vi "test Read Message (TCP) Retries Until Success.vi"(8 "error in (no error)":errorcluster, 11 "TestCase in":refnum<class "TCP API Tests.lvclass">) -> (0 "error out":errorcluster, 3 "TestCase out":refnum<class "TCP API Tests.lvclass">)   [LabVIEW 2013, in "TCP API Tests.lvclass"]
uses:
  TCP API Tests.lvclass
  vi.lib/NI/STM/TCP/TCP Data Info.ctl
  vi.lib/NI/STM/TCP/TCP Read Options.ctl
  vi.lib/NI/STM/TCP/TCP Write Options.ctl
  vi.lib/NI/STM/TCP/Write Meta Data (TCP Ref).vi
  vi.lib/NI/STM/TCP/Read Meta Data (TCP Ref).vi
  vi.lib/NI/STM/TCP/Write Message (TCP).vi
  vi.lib/NI/STM/TCP/Write Meta Data (TCP Clst).vi
  vi.lib/NI/STM/TCP/Read Meta Data (TCP Clst).vi
  vi.lib/NI/STM/TCP/Read Message (TCP).vi
  <vilib>/addons/_JKI Toolkits/VI Tester/TestCase.llb/TestCase.lvclass
  vi.lib/NI/STM/NI STM.lvlib
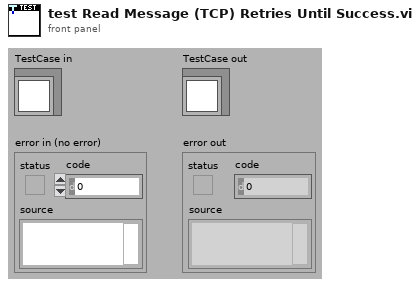
[diagram p1: front panel]
types:
  T1 = typedef "NI STM.lvlib/TCP Data Info.ctl" = cluster{"data size":i32, "retry read":bool}
  T2 = typedef "NI STM.lvlib/TCP Read Options.ctl" = cluster{"ignore timeout error":bool, "timeout ms (1000)":i32}
  T3 = typedef "NI STM.lvlib/TCP Write Options.ctl" = cluster{"ignore timeout error":bool, "timeout ms (1000)":i32}
  T4 = typedef "NI STM.lvlib/TCP Connection Info.ctl" = cluster{"connection ID":refnum<k5>, "meta data":T5[]}
  T5 = typedef "NI STM.lvlib/MetaDataElement.ctl" = string
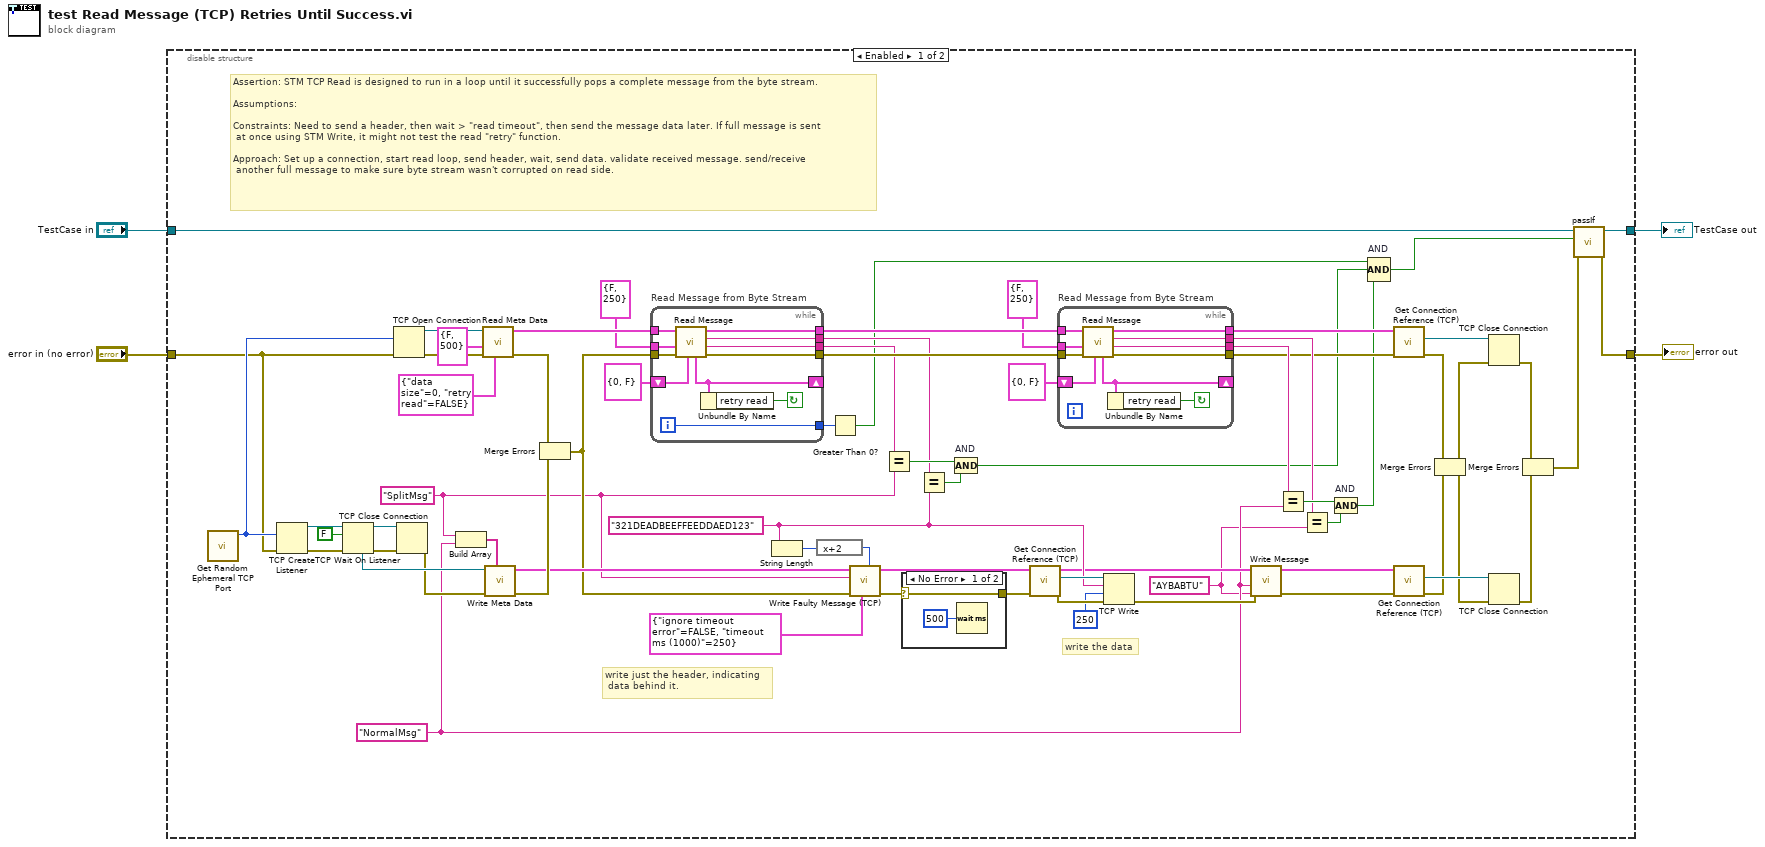
[diagram p0: block diagram]
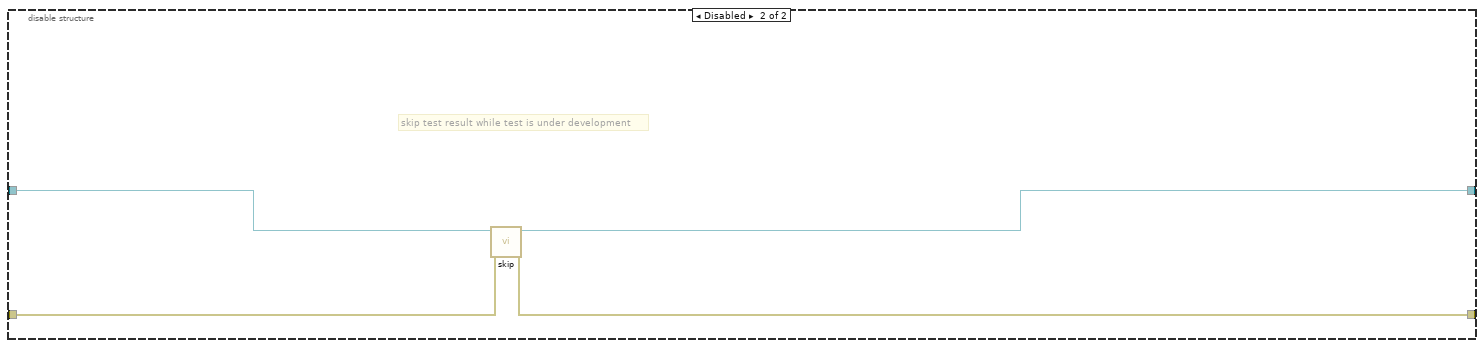
[diagram p3: hidden frame]
diagram:
  n1 = disable-structure shown="Enabled" {
    disable-tunnel: "TestCase in" -> [w72 w100]
    disable-tunnel: [w71 w98] -> w1
    disable-tunnel: [w70 w99] -> w3
    disable-tunnel: "error in (no error)" -> [w56 w97]
    frame Enabled {
      w25 = "AYBABTU" ("data")
      w26 = "NormalMsg" ("Meta Element")
      w39 = "321DEADBEEFFEEDDAED123"
      w40 = "SplitMsg" ("Meta Element")
      # "write the data"
      # "write just the header, indicating\n data behind it."
      # "Assertion: STM TCP Read is designed to run in a loop until it successfully pops a complete message from the byte stream. \n\nAssumptions: \n\nConstraints: Need to send a header, then wait > \"read timeout\", then send the message data later. If full message is sent\n at once using STM Write, it might not test the read \"retry\" function.\n\nApproach: Set up a connection, start read loop, send header, wait, send data. validate received message. send/receive\n another full message to make sure byte stream wasn't corrupted on read side."
      n2 = call "Get Random Ephemeral TCP Port.vi"() -> ("ephemeral TCP port"=w58:u16)  [unwired: 11 in]
      n3 = TCP Create Listener(8:w56, 10:w58) -> (0:w62:errorcluster, 3:w61:refnum<k5>)  [unwired: 3 in, 1 out]
      n4 = TCP Wait On Listener(8:w62, 10:FALSE, 11:w61) -> (0:w63:errorcluster, 3:w60:refnum<k5>, 4:w59:refnum<k5>)  [unwired: 1 in, 2 out]
      n5 = TCP Open Connection(remote port or service name=w58, error in (no error)=w56) -> (connection ID=w69:refnum<k5>, error out=w67:errorcluster)  [unwired: 3 in]
      n6 = TCP Close Connection(connection ID=w60, error in (no error)=w63) -> (error out=w55:errorcluster)  [unwired: 1 in, 1 out]
      n7 = Build Array(w40, w26) -> (w65:string[])
      n8 = call-poly "Read Meta Data.vi"("prev data info"=T1 {"data size"=0, "retry read"=FALSE}, "error in"=w67, "options"=T2 {"ignore timeout error"=FALSE, "timeout ms (1000)"=500}, "connection ID"=w69) -> ("error out"=w68:errorcluster, "connection info out"=w49:T4)  [unwired: 6 out]
      n9 = call-poly "Write Meta Data.vi"("meta data"=w65, "error in"=w55, "connection ID"=w59) -> ("error out"=w66:errorcluster, "connection info out"=w53:T4)  [unwired: 2 in, 5 out]
      n10 = Merge Errors(w68, w66) -> (w50:errorcluster)
      n11 = while "Read Message from Byte Stream" {
        tunnel: w49 -> [w96]
        tunnel: w50 -> [w95]
        tunnel: [w94] -> w28
        tunnel: [w93] -> w29
        tunnel: [w89] -> w33
        tunnel: [w92] -> w34
        shift-right: [w90] -> _
        shift-left: T1 {"data size"=0, "retry read"=FALSE} ("data info") -> [w91]
        tunnel: T2 {"ignore timeout error"=FALSE, "timeout ms (1000)"=250} ("options") -> [w88]
        tunnel: [w86] -> w6
        i -> [w86]
        stop <- w87 continue-if-true
        n12 = call-poly "Read Message.vi"("prev data info"=w91, "error in"=w95, "options"=w88, "connection info in"=w96) -> ("error out"=w89:errorcluster, "name"=w94:T5, "data string"=w93:string, "connection info out"=w92:T4, "data info"=w90:T1)  [unwired: 1 in, 2 out]
        n13 = Unbundle By Name(w90) -> ("retry read"=w87:bool)
      }
      n14 = String Length(string=w39) -> (length=w42:i32)
      n15 = expression code="x+2"(w42) -> (w7:i32)
      n16 = Greater Than 0?(x=w6) -> (x > 0?=w5:bool)
      n17 = call "Write Faulty Message (TCP).vi"("total message length [B] (-1: calculate)"=w7, "options"=T3 {"ignore timeout error"=FALSE, "timeout ms (1000)"=250}, "error in"=w50, "name (\"\")"=w40, "connection info in"=w53) -> ("error out"=w47:errorcluster, "connection info out"=w44:T4)  [unwired: 5 in]
      n18 = Equal?(x=w28, y=w40) -> (x = y?=w38:bool)
      n19 = case shown="No Error" w47 {
        selector: w47 -> [w83 w85]
        tunnel: [w83 w85] -> w46
        frame No Error {
          n20 = Wait (ms)(milliseconds to wait=u32 500) -> ()  [unwired: 1 out]
        }
        frame Error {
        }
      }
      n21 = Equal?(x=w29, y=w39) -> (x = y?=w37:bool)
      n22 = Compound Arithmetic op=AND "AND"(w38, w37) -> (w17:bool)
      n23 = call "Get Connection Reference (TCP).vi"("error in"=w46, "connection info in"=w44) -> ("error out"=w45:errorcluster, "connection ID out"=w43:refnum<k5>, "connection info out"=w36:T4)  [unwired: 7 in]
      n24 = while "Read Message from Byte Stream" {
        tunnel: w34 -> [w82]
        tunnel: w33 -> [w81]
        tunnel: [w80] -> w27
        tunnel: [w79] -> w24
        tunnel: [w75] -> w22
        tunnel: [w78] -> w23
        shift-right: [w76] -> _
        shift-left: T1 {"data size"=0, "retry read"=FALSE} ("data info") -> [w77]
        tunnel: T2 {"ignore timeout error"=FALSE, "timeout ms (1000)"=250} ("options") -> [w74]
        stop <- w73 continue-if-true
        n25 = call-poly "Read Message.vi"("prev data info"=w77, "error in"=w81, "options"=w74, "connection info in"=w82) -> ("error out"=w75:errorcluster, "name"=w80:T5, "data string"=w79:string, "connection info out"=w78:T4, "data info"=w76:T1)  [unwired: 1 in, 2 out]
        n26 = Unbundle By Name(w76) -> ("retry read"=w73:bool)
      }
      n27 = TCP Write(connection ID=w43, data in=w39, error in (no error)=w45, 9:250 ("timeout ms (25000)")) -> (error out=w35:errorcluster)  [unwired: 2 out]
      n28 = call-poly "Write Message.vi"("error in"=w35, "data"=w25, "name"=w26, "connection info in"=w36) -> ("error out"=w20:errorcluster, "connection info out"=w21:T4)  [unwired: 6 in]
      n29 = Equal?(x=w27, y=w26) -> (x = y?=w30:bool)
      n30 = Equal?(x=w24, y=w25) -> (x = y?=w31:bool)
      n31 = Compound Arithmetic op=AND "AND"(w30, w31) -> (w16:bool)
      n32 = Compound Arithmetic op=AND "AND"(w5, w17, w16) -> (w15:bool)
      n33 = call "Get Connection Reference (TCP).vi"("error in"=w22, "connection info in"=w23) -> ("error out"=w14:errorcluster, "connection ID out"=w18:refnum<k5>)  [unwired: 7 in, 1 out]
      n34 = call "Get Connection Reference (TCP).vi"("error in"=w20, "connection info in"=w21) -> ("error out"=w13:errorcluster, "connection ID out"=w19:refnum<k5>)  [unwired: 7 in, 1 out]
      n35 = Merge Errors(w14, w13) -> (w12:errorcluster)
      n36 = TCP Close Connection(connection ID=w18, error in (no error)=w12) -> (error out=w11:errorcluster)  [unwired: 1 in, 1 out]
      n37 = TCP Close Connection(connection ID=w19, error in (no error)=w12) -> (error out=w10:errorcluster)  [unwired: 1 in, 1 out]
      n38 = Merge Errors(w11, w10) -> (w9:errorcluster)
      n39 = call-dynamic "passIf.vi"("error in (no error)"=w9, "pass"=w15, "TestCase in"=w72) -> ("error out"=w70:errorcluster, "TestCase out"=w71:refnum<class "TCP API Tests.lvclass">)  [unwired: 7 in]
    }
    frame Disabled {
      # "skip test result while test is under development"
      n40 = call <vilib>:"skip.vi"("error in (no error)"=w97, "TestCase in"=w100) -> ("error out"=w99:errorcluster, "TestCase out"=w98:refnum<class "TCP API Tests.lvclass">)  [unwired: 8 in]
    }
  }
  "error out" <- w3
  "TestCase out" <- w1
